vi "Lab_Wrapper.vi"(8 "error in (no error)":errorcluster, 11 "Input Array":variant[](array[variant])) -> (0 "error out":errorcluster, 3 "Output Array":variant[](array[variant]))   [LabVIEW 2013]
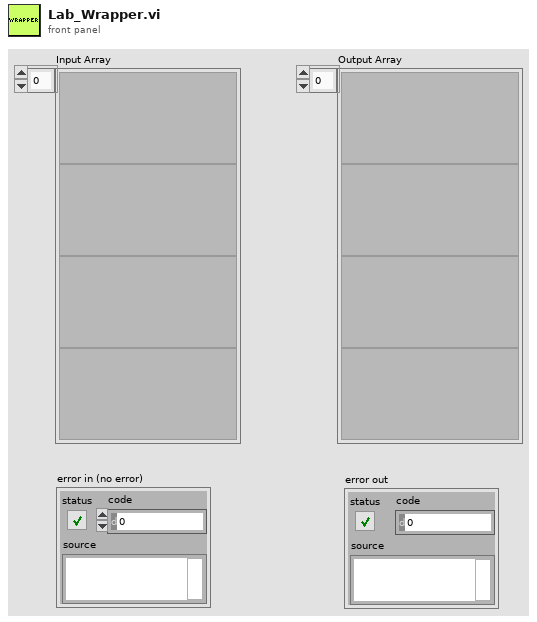
[diagram p1: front panel]
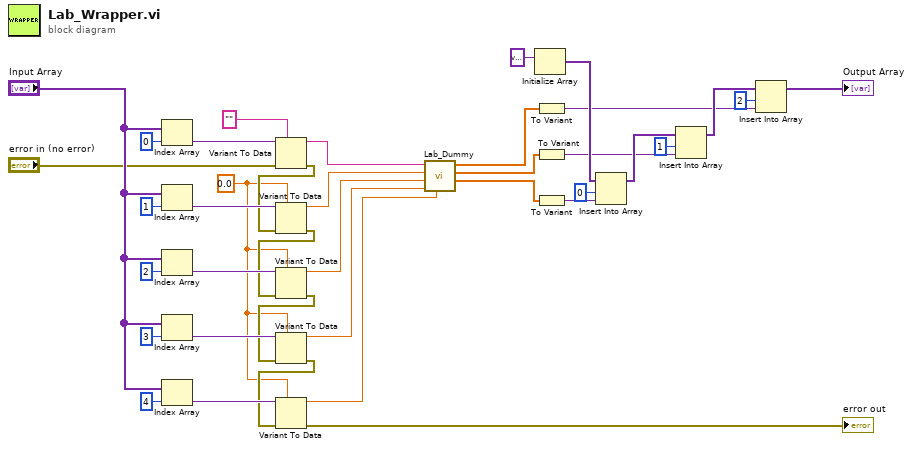
[diagram p0: block diagram]
diagram:
  w1 = 0.0
  n1 = Index Array(array="Input Array", index=0) -> (element=w24:variant)
  n2 = Index Array(array="Input Array", index=1) -> (element=w23:variant)
  n3 = Index Array(array="Input Array", index=2) -> (element=w22:variant)
  n4 = Index Array(array="Input Array", index=3) -> (element=w21:variant)
  n5 = Index Array(array="Input Array", index=4) -> (element=w20:variant)
  n6 = Variant To Data(error in="error in (no error)", type="", Variant=w24) -> (data=w7:string, error out=w18:errorcluster)
  n7 = Variant To Data(error in=w18, type=w1, Variant=w23) -> (data=w6:dbl, error out=w17:errorcluster)
  n8 = Variant To Data(error in=w17, type=w1, Variant=w22) -> (data=w5:dbl, error out=w16:errorcluster)
  n9 = Variant To Data(error in=w16, type=w1, Variant=w21) -> (data=w4:dbl, error out=w15:errorcluster)
  n10 = Variant To Data(error in=w15, type=w1, Variant=w20) -> (data=w3:dbl, error out=→"error out":errorcluster)
  n11 = call "Lab_Dummy.vi"("Unused Input 5"=w3, "Unused Input 4"=w4, "Unused Input 3"=w5, "Unused Input 2"=w6, "Unused Input 1"=w7) -> ("Time"=w27:dbl[], "Vout"=w28:dbl[], "Vin"=w26:dbl[])  [unwired: 4 in]
  n12 = Initialize Array(variant ("variant")) -> (w38:variant[])  [unwired: 1 in]
  n13 = To Variant(anything=w26) -> (Variant=w29:variant)
  n14 = To Variant(anything=w28) -> (Variant=w30:variant)
  n15 = To Variant(anything=w27) -> (Variant=w31:variant)
  n16 = Insert Into Array(array=w38, index=0, new element=w31) -> (w36:variant[])
  n17 = Insert Into Array(array=w36, index=1, new element=w30) -> (w37:variant[])
  n18 = Insert Into Array(array=w37, index=2, new element=w29) -> (→"Output Array":variant[])
